vi "Match.vi"() -> ()   [LabVIEW 2024]
panel:
  in  "stop":bool
  out "Iteration Count":i32
  in  "Number to Match":dbl
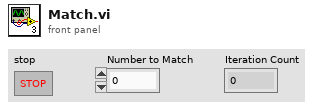
[diagram p1: front panel]
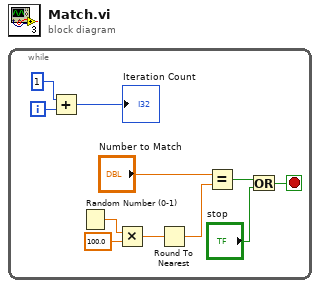
[diagram p0: block diagram]
diagram:
  n1 = while {
    i -> [w6]
    stop <- w4 stop-if-true
    n2 = Add(x=1, y=w6) -> (x+y=→"Iteration Count":i32)
    n3 = Random Number (0-1)() -> (number: 0 to 1=w9:dbl)
    n4 = Multiply(x=w9, y=100.0) -> (x*y=w10:dbl)
    n5 = Round To Nearest(number=w10) -> (nearest integer value=w11:dbl)
    n6 = Equal?(x="Number to Match", y=w11) -> (x = y?=w3:bool)
    n7 = Or(x=w3, y="stop") -> (x .or. y?=w4:bool)
  }
